vi "FG-Configuration.vi"(8 "error in":errorcluster, 9 "Acquis. params. ref.":refnum<data-value>, 10 "Storage params in":refnum<data-value>, 11 "Config. params. ref.":refnum<data-value>) -> (0 "error IO":errorcluster, 2 "Storage params":refnum<data-value>, 3 "Config. params. ref.":refnum<data-value>, 5 "Succes?":bool)   [LabVIEW 2013, in "CameraVision.lvlib" / "CV-Configuration.lvclass"]
uses:
  CV-Configuration.lvclass
  Acquisition/CV-Acquisition.lvclass
  Storage/CV-Storage.lvclass
  Storage/CV-Storage.lvclass/CV-Storage.ctl
  CV-Configuration.lvclass/CV-Configuration.ctl
  UI/Popup-messages.ctl
  Storage/Read Base path.vi
  Read Camera config file.vi
  UI/CV-UI.lvclass
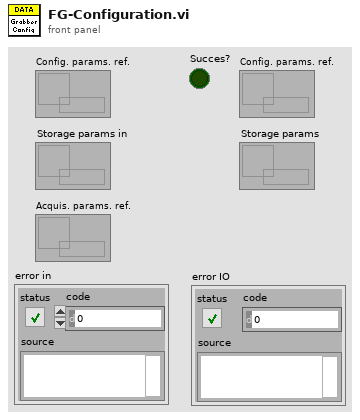
[diagram p1: front panel]
types:
  T1 = enum16{"open", "replace", "create", "open or create", "replace or create", "replace or create with confirmation"}
  T2 = typedef "CameraVision.lvlib/CV-UI.lvclass/Popup-messages.ctl" = enum16{"Error-Black image", "Error-Camera config file", "Error-Camera connect", "Error-Grabber init", "Error-Camera setting", "Error-Image offset", "Error-Image import", "Error-Settings file not exist", "Error-Timing source", "Conflict-Filters", "Conflict-Map", "Conflict-Framerate", "Conflict-Charact", "Conflict-Temperature field", "Conflict-Temperature value", "Conflict-Storage-Binary image", "Conflict-Storage-Corrected image", "Conflict-Storage-Map", "Conflict-Storage-Charact", "Conflict-Storage-Temperature field", "Conflict-Storage-Temperature value", "Warning-File exist", "Warning-Parameter reset", "Warning-User cancel", "Info-Images imported"}
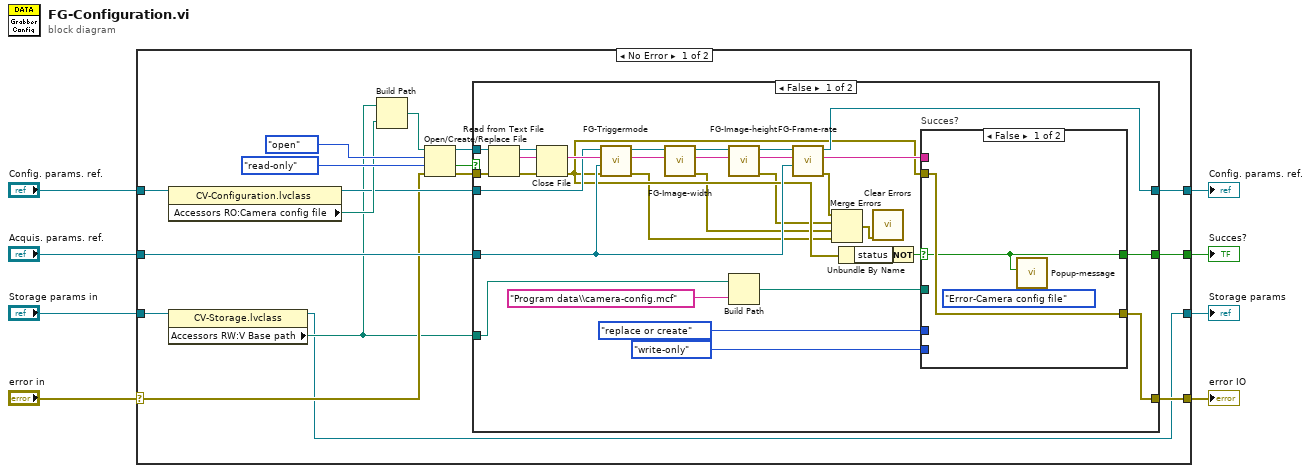
[diagram p0: block diagram]
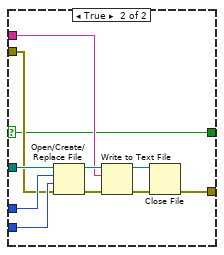
[diagram p2: hidden frame]
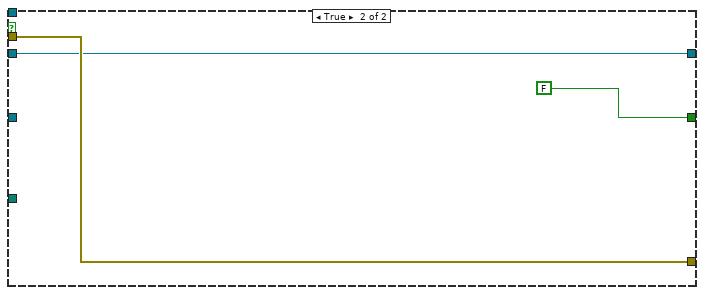
[diagram p3: hidden frame]
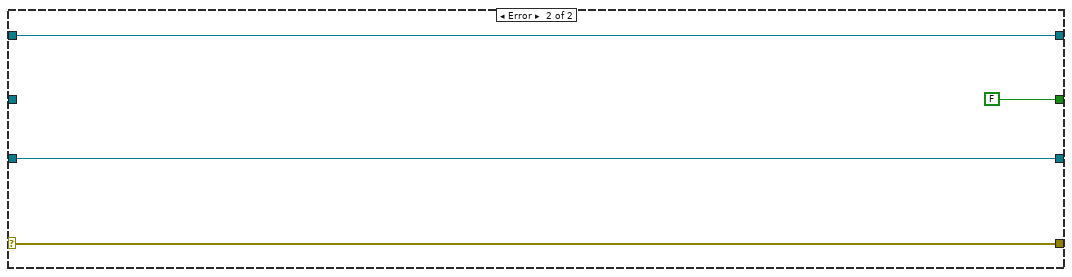
[diagram p4: hidden frame]
diagram:
  n1 = case shown="No Error" "error in" {
    selector: "error in" -> [w12 w76]
    tunnel: [w25 w76] -> w8
    tunnel: "Config. params. ref." -> [w18 w74]
    tunnel: [w19 FALSE] -> w7
    tunnel: "Acquis. params. ref." -> [w14 _]
    tunnel: [w13 w74] -> w3
    tunnel: "Storage params in" -> [w11 w73]
    tunnel: [w9 w73] -> w1
    frame No Error {
      n2 = property class="CV-Configuration.lvclass"(reference=w18) -> (reference out=w15:refnum<data-value>, "Accessors RO:Camera config file"=w16:path)  [unwired: 1 in, 1 out]
      n3 = property class="CV-Storage.lvclass"(reference=w11) -> (reference out=w9:refnum<data-value>, "Accessors RW:V Base path"=w10:path)  [unwired: 1 in, 1 out]
      n4 = Build Path(base path=w10, name or relative path=w16) -> (appended path=w17:path)
      n5 = Open/Create/Replace File(file path (use dialog)=w17, error in=w12, operation (0:open)=T1."open", access (0:read/write)=enum16{"read/write", "read-only", "write-only"}."read-only") -> (refnum out=w22:refnum<file>, cancelled=w23:bool, error out=w24:errorcluster)  [unwired: 2 in]
      n6 = case shown="False" w23 {
        tunnel: w22 -> [w55 _]
        tunnel: w24 -> [w51 w71]
        tunnel: [w48 w71] -> w25
        tunnel: [w47 FALSE] -> w19
        tunnel: w15 -> [w42 w70]
        tunnel: w14 -> [w38 _]
        tunnel: [w34 w70] -> w13
        tunnel: w10 -> [w26 _]
        frame False {
          n7 = Read from Text File(file (use dialog)=w55, error in=w51) -> (refnum out=w54:refnum<file>, text=w43:string, error out=w53:errorcluster)  [unwired: 2 in, 1 out]
          n8 = Close File(refnum=w54, error in=w53) -> (error out=w32:errorcluster)  [unwired: 1 out]
          n9 = call "FG-Triggermode.vi"("error in"=w32, "Acquis. params. ref."=w38, "Config file string in"=w43, "Config. params. ref. in"=w42) -> ("error IO"=w27:errorcluster, "Config file string"=w41:string, "Config. params. ref."=w40:refnum<data-value>)  [unwired: 4 in, 1 out]
          n10 = call "FG-Image-width.vi"("Config file string in"=w41, "Config. params. ref. in"=w40) -> ("error IO"=w28:errorcluster, "Config file string"=w45:string, "Config. params. ref."=w39:refnum<data-value>)  [unwired: 6 in, 1 out]
          n11 = call "FG-Image-height.vi"("Config file string in"=w45, "Config. params. ref. in"=w39) -> ("error IO"=w29:errorcluster, "Config file string"=w44:string, "Config. params. ref."=w37:refnum<data-value>)  [unwired: 6 in, 1 out]
          n12 = Build Path(base path=w26, name or relative path="Program data\\camera-config.mcf") -> (appended path=w46:path)
          n13 = call "FG-Frame-rate.vi"("Acquis. params. ref."=w38, "Config file string in"=w44, "Config. params. ref. in"=w37) -> ("error IO"=w30:errorcluster, "Config file string"=w36:string, "Config. params. ref."=w34:refnum<data-value>)  [unwired: 5 in, 1 out]
          n14 = Merge Errors(w30, w29, w28, w27) -> (w31:errorcluster)
          n15 = Unbundle By Name(w32) -> ("status"=w35:bool)
          n16 = call <vilib>:"Clear Errors.vi"("error in (no error)"=w31) -> ()  [unwired: 6 in, 1 out]
          n17 = Not(x=w35) -> (.not. x?=w33:bool)
          n18 = case "Succes?" shown="False" w33 {
            selector: w33 -> [w56 w59]
            tunnel: w46 -> [_ w65]
            tunnel: T1."replace or create" ("operation (0:open)") -> [_ w64]
            tunnel: enum16{"read/write", "read-only", "write-only"}."write-only" ("access (0:read/write)") -> [_ w63]
            tunnel: [w58 w62] -> w48
            tunnel: [w56 w59] -> w47
            tunnel: w36 -> [_ w61]
            tunnel: w32 -> [w58 w60]
            frame False {
              n19 = call "Popup-message.vi"("Message"=Popup-messages."Error-Camera config file", "Ignore?"=w56) -> ()  [unwired: 9 in, 1 out]
            }
            frame True {
              n20 = Open/Create/Replace File(file path (use dialog)=w65, error in=w60, operation (0:open)=w64, access (0:read/write)=w63) -> (refnum out=w69:refnum<file>, error out=w66:errorcluster)  [unwired: 2 in, 1 out]
              n21 = Write to Text File(file (use dialog)=w69, text=w61, error in=w66) -> (refnum out=w68:refnum<file>, error out=w67:errorcluster)  [unwired: 1 in, 1 out]
              n22 = Close File(refnum=w68, error in=w67) -> (error out=w62:errorcluster)  [unwired: 1 out]
            }
          }
        }
        frame True {
        }
      }
    }
    frame Error {
    }
  }
  "error IO" <- w8
  "Succes?" <- w7
  "Config. params. ref." <- w3
  "Storage params" <- w1
